vi "Angular PID Global.vi"() -> ()   [LabVIEW 2015]
panel:
  in  "Current Encoder Position":dbl
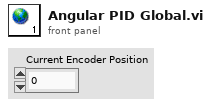
[diagram p1: front panel]
diagram:
